vi "MoveBaxterArms.vi"(2 "node":string, 3 "Parameters":T1 {"left_w2" scale=-180.0..180.0; "left_w1" scale=-180.0..180.0; "left_w0" scale=-180.0..180.0; "left_e1" scale=-180.0..180.0; "left_e0" scale=-180.0..180.0; "left_s1" scale=-180.0..180.0; "left_s0" scale=-180.0..180.0; "right_s1" scale=-180.0..180.0; "right_s0" scale=-180.0..180.0; "right_w2" scale=-180.0..180.0; "right_e1" scale=-180.0..180.0; "right_e0" scale=-180.0..180.0; "right_w0" scale=-180.0..180.0; "right_w1" scale=-180.0..180.0}, 6 "error in":errorcluster) -> (5 "error out":errorcluster)   [LabVIEW 2010]
doc: "This VI moves both the Baxter arms to a given position."
uses:
  <userlib>/ROSforLV_0.1/ROS/Code/JointPositions.ctl
  <userlib>/ROSforLV_0.1/ROS/Code/Slider.ctl
  <userlib>/ROSforLV_0.1/ROS/Code/SubVIs/BaxterSide.ctl
panel:
  # "If Stop Cont is set to true, the server will\nstop continuously writing"
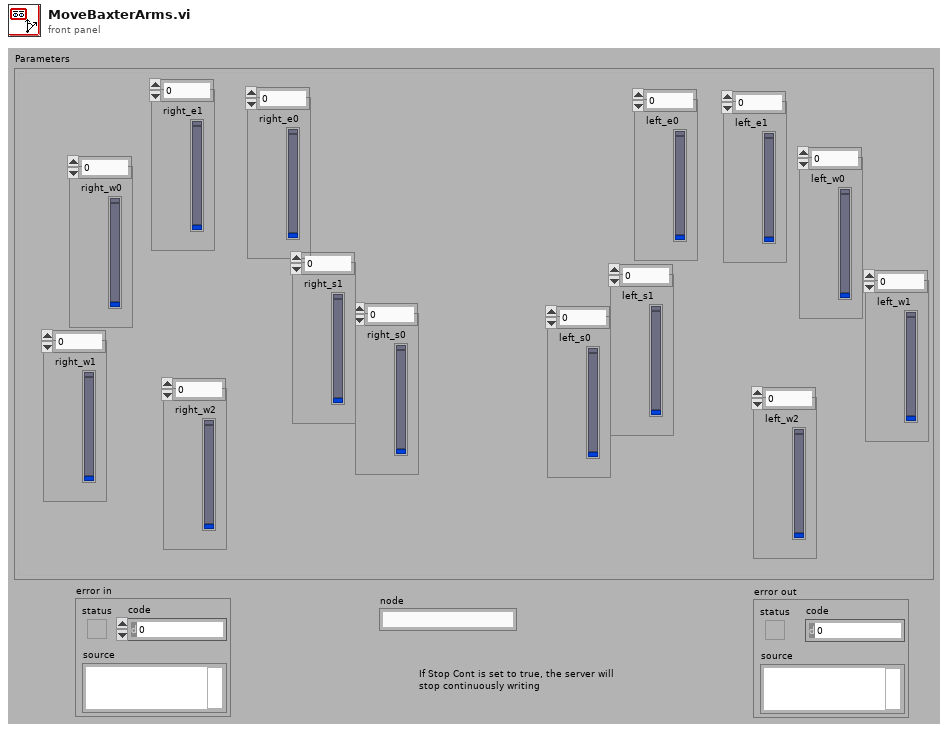
[diagram p1: front panel]
types:
  T1 = typedef "JointPositions.ctl" = cluster{"left_e0":T2, "left_e1":T2, "left_s0":T2, "left_s1":T2, "left_w0":T2, "left_w1":T2, "left_w2":T2, "right_e0":T2, "right_e1":T2, "right_s0":T2, "right_s1":T2, "right_w0":T2, "right_w1":T2, "right_w2":T2}
  T2 = typedef "Slider.ctl" = dbl
  T3 = typedef "BaxterSide.ctl" = enum16{"left", "right"}
  T4 = cluster{"[0]":T2, "[1]":T2, "[2]":T2, "[3]":T2, "[4]":T2, "[5]":T2, "[6]":T2}
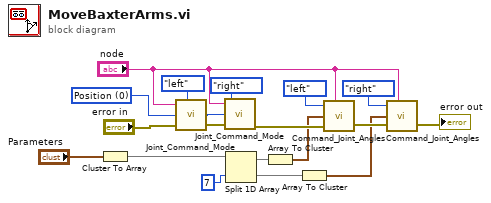
[diagram p0: block diagram]
diagram:
  w11 = u8 0 items=["Position", "Velocity", "Effort"] ("Mode")
  n1 = Cluster To Array(cluster="Parameters") -> (array=w1:T2[])
  n2 = call <userlib>:"Joint_Command_Mode.vi"("Side"=BaxterSide."left", "node"="node", "Mode"=w11, "error in"="error in") -> ("error out"=w13:errorcluster)  [unwired: 2 in]
  n3 = call <userlib>:"Joint_Command_Mode.vi"("Side"=BaxterSide."right", "node"="node", "Mode"=w11, "error in"=w13) -> ("error out"=w12:errorcluster)  [unwired: 2 in]
  n4 = Split 1D Array(array=w1, index=7) -> (first subarray=w5:T2[], second subarray=w4:T2[])
  n5 = Array To Cluster(array=w5) -> (cluster=w3:T4)
  n6 = Array To Cluster(array=w4) -> (cluster=w2:T4)
  n7 = call <userlib>:"Command_Joint_Angles.vi"("Side"=BaxterSide."left", "node"="node", "Arm Angles (degrees)"=w3, "error in"=w12) -> ("error out"=w15:errorcluster)  [unwired: 2 in]
  n8 = call <userlib>:"Command_Joint_Angles.vi"("Side"=BaxterSide."right", "node"="node", "Arm Angles (degrees)"=w2, "error in"=w15) -> ("error out"=→"error out":errorcluster)  [unwired: 2 in]
